vi "Clone.vi"(8 "error in":errorcluster, 11 "Cell View in":refnum<class "Cell View.lvclass">) -> (0 "error out":errorcluster, 2 "Clone":refnum<class "Cell View.lvclass">, 3 "Cell View out":refnum<class "Cell View.lvclass">)   [LabVIEW 2023, in "SourceGrid.lvlib" / "Cell View.lvclass"]
uses:
  Cell View.lvclass
  Cell View.lvclass/Cell View.ctl
  D:/git/Sourcegrid-LabVIEW/dll/SourceGrid.dll
  dll/SourceGrid.dll
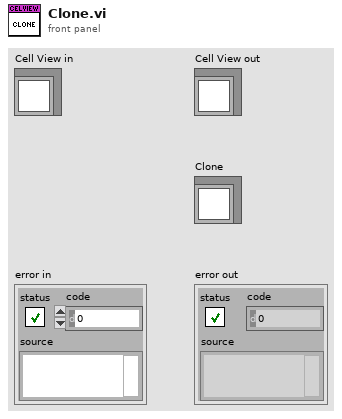
[diagram p1: front panel]
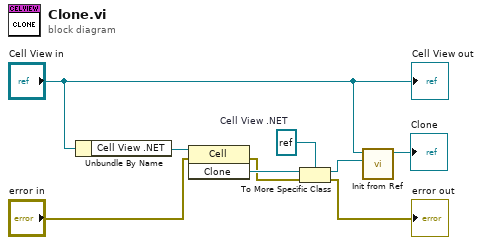
[diagram p0: block diagram]
diagram:
  w4 = refnum<k24> refnum  # Cell View .NET
  n1 = Unbundle By Name("Cell View in") -> ("Cell View .NET"=w9:refnum<k24>)
  n2 = invoke class="Cell" method="Clone"(reference=w9, error in="error in") -> (error out=w6:errorcluster, "Clone"=w7:refnum<k24>)  [unwired: 1 in, 1 out]
  n3 = To More Specific Class(target class=w4, reference=w7, error in=w6) -> (specific class reference=w3:refnum<k24>, error out=→"error out":errorcluster)
  n4 = call-dynamic "Init from Ref.vi"("Cell View .NET"=w3, "Cell View in"="Cell View in") -> ("Cell View out"=→"Clone":refnum<class "Cell View.lvclass">)  [unwired: 9 in]
  "Cell View out" <- "Cell View in"
